vi "IR_Sensor_Test.vi"() -> ()   [LabVIEW 2014]
uses:
  <vilib>/eio/EIONode/EIONode.xnode
  <vilib>/rvi/Analysis/measure/butterworth/XNode/niFpgaButterworthFilter.xnode
  <vilib>/rvi/eio/common/nirviEmuTemplateMethod_errors.vi
panel:
  in  "stop ball":bool
  in  "Frequency (kHz)":u32
  in  "Duty Cycle (%)":u32
  in  "stop":bool
  out "Waveform Chart":sgl(graph)
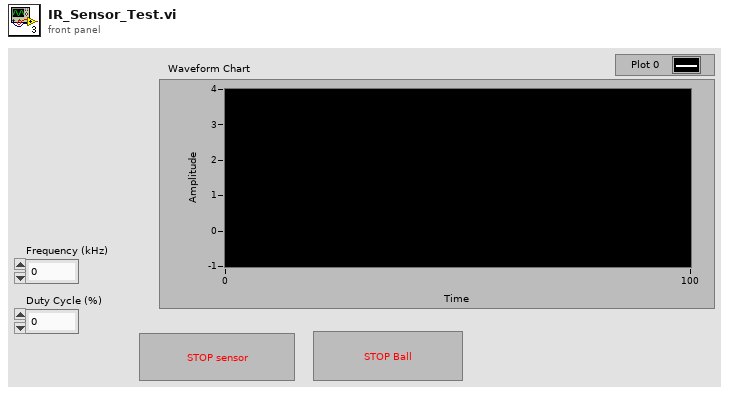
[diagram p1: front panel]
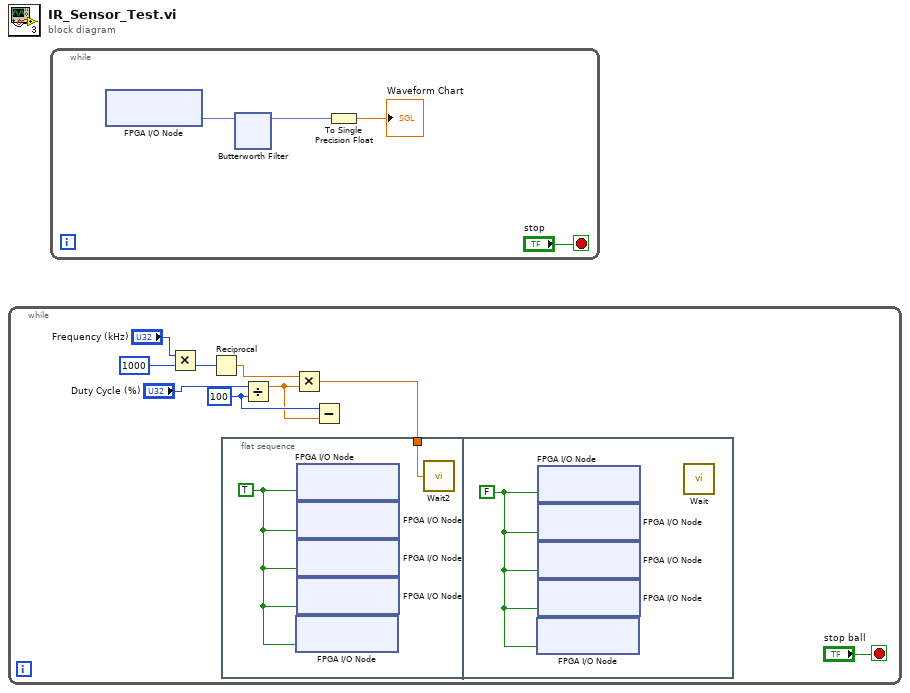
[diagram p0: block diagram]
diagram:
  n1 = while {
    stop <- "stop ball" stop-if-true
    w4 = u32 100 ("y")
    n2 = Multiply(x="Frequency (kHz)", y=u32 1000 ("x")) -> (x*y=w2:u32)
    n3 = Reciprocal(x=w2) -> (1/x=w7:dbl)
    n4 = flat-sequence {
      tunnel: w5 -> [w10]
      frame #0 {
        w11 = TRUE ("DO0")
        n5 = xnode "FPGA I/O Node"("Mod3/DO4"=w11) -> ()  [unwired: 1 in, 1 out]
        n6 = xnode "FPGA I/O Node"("Mod3/DO0"=w11) -> ()  [unwired: 1 in, 1 out]
        n7 = xnode "FPGA I/O Node"("Mod3/DO1"=w11) -> ()  [unwired: 1 in, 1 out]
        n8 = xnode "FPGA I/O Node"("Mod3/DO2"=w11) -> ()  [unwired: 1 in, 1 out]
        n9 = xnode "FPGA I/O Node"("Mod3/DO3"=w11) -> ()  [unwired: 1 in, 1 out]
        n10 = call "Wait2"("Count(uSec)"=w10) -> ()  [unwired: 1 out]
      }
      frame #1 {
        w12 = FALSE ("DO0")
        n11 = xnode "FPGA I/O Node"("Mod3/DO4"=w12) -> ()  [unwired: 1 in, 1 out]
        n12 = xnode "FPGA I/O Node"("Mod3/DO0"=w12) -> ()  [unwired: 1 in, 1 out]
        n13 = xnode "FPGA I/O Node"("Mod3/DO1"=w12) -> ()  [unwired: 1 in, 1 out]
        n14 = xnode "FPGA I/O Node"("Mod3/DO2"=w12) -> ()  [unwired: 1 in, 1 out]
        n15 = xnode "FPGA I/O Node"("Mod3/DO3"=w12) -> ()  [unwired: 1 in, 1 out]
        n16 = call "Wait"() -> ()  [unwired: 1 in, 1 out]
      }
    }
    n17 = Divide(x="Duty Cycle (%)", y=w4) -> (x/y=w3:dbl)
    n18 = Multiply(x=w7, y=w3) -> (x*y=w5:dbl)
    n19 = Subtract(x=w4, y=w3) -> ()  [unwired: 1 out]
  }
  n20 = while {
    stop <- "stop" stop-if-true
    n21 = xnode "FPGA I/O Node"() -> ("Mod2/AI0"=w15:fxp<+/-,16,5>)  [unwired: 1 in, 1 out]
    n22 = xnode "Butterworth Filter"("input data"=w15) -> ("output data"=w14:fxp<+/-,20,9>)  [unwired: 2 in]
    n23 = To Single Precision Float(number=w14) -> (single precision float=→"Waveform Chart":sgl)
  }
